vi "Read Device ID Type Request.vi"(8 "error in (no error)":errorcluster, 9 "object ID":u8, 10 "read device ID code":T1(ring)) -> (0 "error out":errorcluster, 2 "Modbus data unit out":refnum<class "Modbus Data Unit (PDU).lvclass">)   [LabVIEW 2018, in "SubVIs.lvlib" / "Master Function Definition.lvlib"]
doc: "This VI forms the modbus data unit for reading the device identification."
uses:
  Master Function Definition.lvlib
  Modbus Data Unit (PDU).lvclass
  Modbus Data Unit (PDU).lvclass/Modbus Data Unit (PDU).ctl
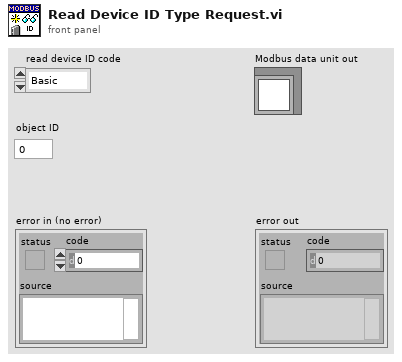
[diagram p1: front panel]
types:
  T1 = enum8{"Basic", "Regular", "Extended", "Specific"}
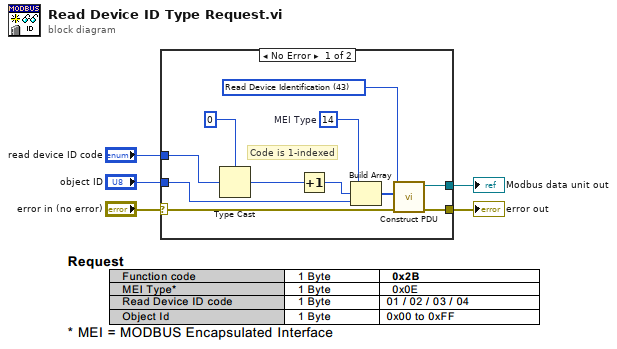
[diagram p0: block diagram]
diagram:
  n1 = case shown="No Error" "error in (no error)" {
    selector: "error in (no error)" -> [w6 w17]
    tunnel: [w16 w17] -> w5
    tunnel: [w15 _] -> w4
    tunnel: "read device ID code" -> [w11 _]
    tunnel: "object ID" -> [w10 _]
    frame No Error {
      w12 = u8 14  # MEI Type
      w13 = u8 43 items=["Read Discrete Inputs"=2, "Read Coils"=1, "Write Single Coil"=5, "Write Multiple Coils"=15, "Read Input Register"=4, "Read Holding Registers"=3, "Write Single Register"=6, "Write Multiple Registers"=16, "Read/Write Multiple Registers"=23, "Mask Write Register"=22, "Read FIFO Queue"=24, "Read File Record"=20, "Write File Record"=21, "Read Exception Status"=7, "Diagnostic"=8, "Get Com Event Counter"=11, "Get Com Event Log"=12, "Report Slave ID"=17, "Read Device Identification"=43] ("Function")
      # "Code is 1-indexed"
      n2 = Type Cast(type=u8 0 ("MEI Type 2"), x=w11) -> (*(type *) &x=w9:u8)
      n3 = Increment ("Code is 1-indexed")(x=w9) -> (x+1=w7:u8)
      n4 = Build Array(w12, w7, w10) -> (w14:u8[])
      n5 = call "Construct PDU.vi"("error in (no error)"=w6, "data"=w14, "function"=w13) -> ("error out"=w16:errorcluster, "Modbus data unit out"=w15:refnum<class "Modbus Data Unit (PDU).lvclass">)  [unwired: 7 in]
    }
    frame Error {
    }
  }
  "error out" <- w5
  "Modbus data unit out" <- w4
